vi "Globals.vi"() -> ()   [LabVIEW 2015]
panel:
  out "slide":i32
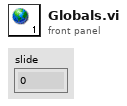
[diagram p1: front panel]
diagram:
